vi "Element Events.vi"(8 "error in (no error)":errorcluster, 11 "LoggingControl in":refnum<class "LoggingControl.lvclass">) -> (0 "error out":errorcluster, 2 "Element Events":refnum<class "Control Event Registrations.lvclass">, 3 "LoggingControl out":refnum<class "LoggingControl.lvclass">)   [LabVIEW 2020, in "VolatusGUIElements.lvlib" / "LoggingControl.lvclass"]
uses:
  LoggingControl.lvclass
  C:/dev/lv20CE/relink/lv-volatus/VolatusGUI/OnValueChangeHandler/OnValueChangeHandler.lvclass
  VolatusGUI/Control Event Registrations/Control Event Registrations.lvclass
  LoggingControl.lvclass/LoggingControl.ctl
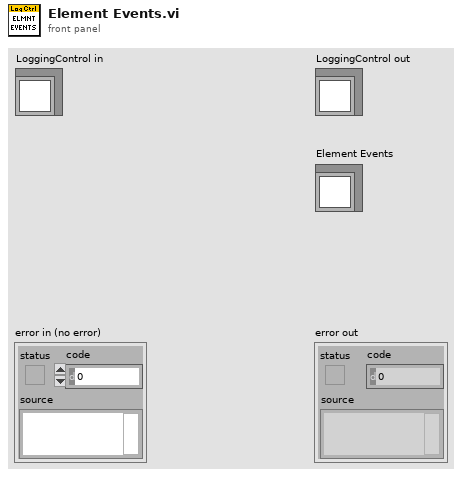
[diagram p1: front panel]
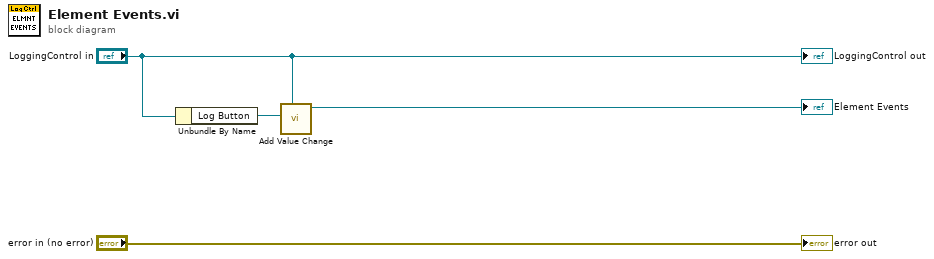
[diagram p0: block diagram]
diagram:
  n1 = Unbundle By Name("LoggingControl in") -> ("Log Button"=w3:refnum<vi>)
  n2 = call "Add Value Change.vi"("Control"="LoggingControl in", "CtlRef"=w3) -> ("Control Event Registrations out"=→"Element Events":refnum<class "Control Event Registrations.lvclass">)  [unwired: 8 in, 1 out]
  "error out" <- "error in (no error)"
  "LoggingControl out" <- "LoggingControl in"
